vi "Employee_Lookup(py).vi"(0 "Badge Scan In(str)":string, 11 "error in (no error)":errorcluster, 12 "Enable(t)":bool) -> (2 "standard output":string, 3 "Success?(t)":bool, 15 "error out":errorcluster)   [LabVIEW 2018]
uses:
  <vilib>/Utility/error.llb/DialogType.ctl
  Initialize References/Sequence Globals.vi
panel:
  out "py path":path
  out "Badge Scan Out(str)":string
  in  "ByPass(t)":bool
  out "SwExists?(t)":bool
  out "NameMatch?(t)":bool
  out "BadgeName":string
  out "DbName":string
  out "EmpNumMatch?(t)":bool
  out "DataBaseError?(T)":bool
  out "standard error":string
  # "001, RICK QUINTAL, NBPT"
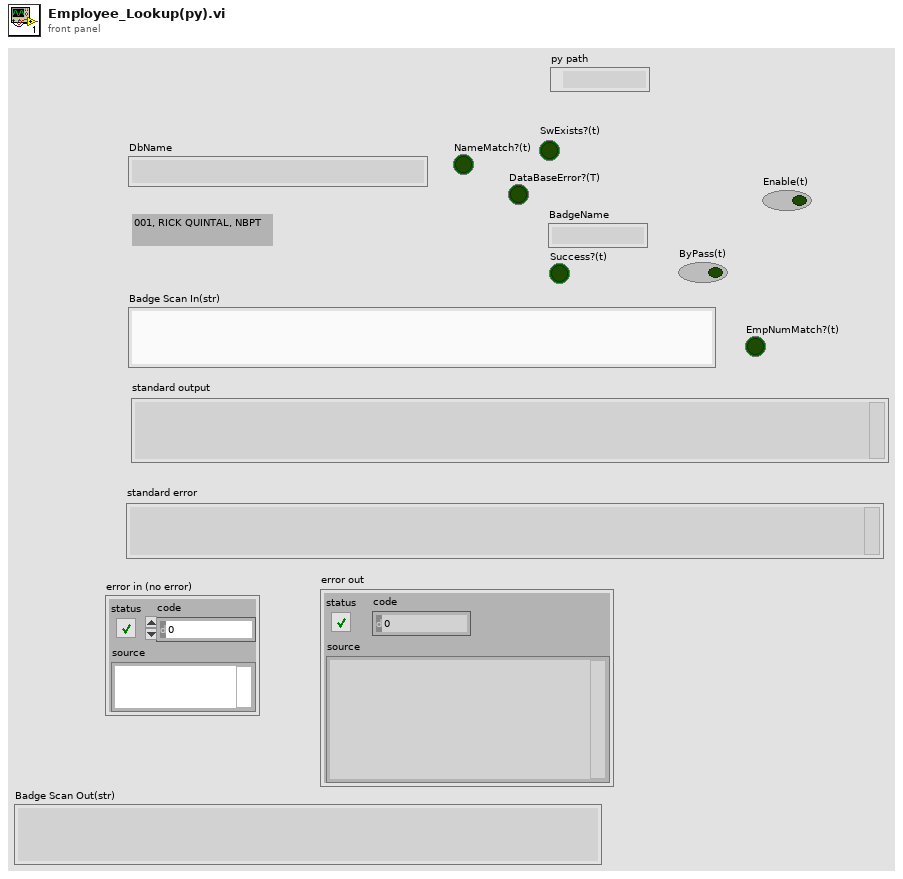
[diagram p1: front panel]
types:
  T1 = typedef "DialogType.ctl" = u16
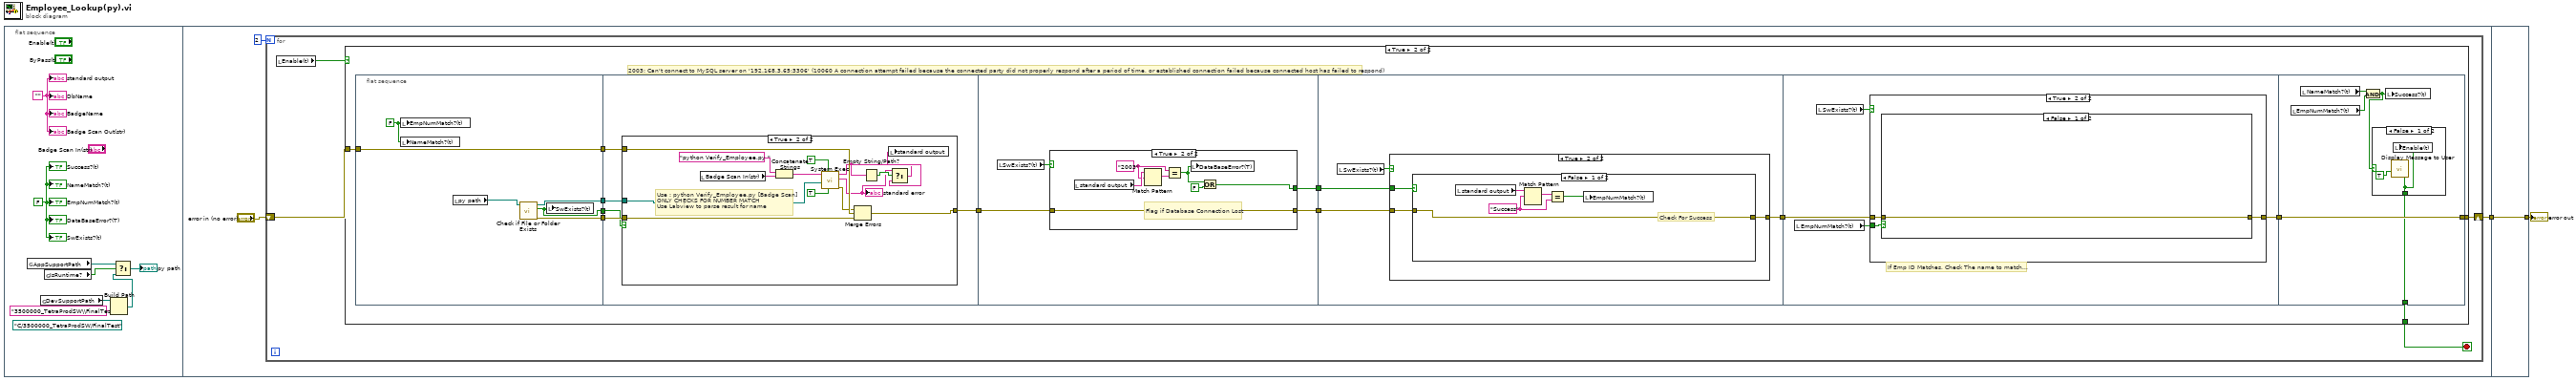
[diagram p0: block diagram]
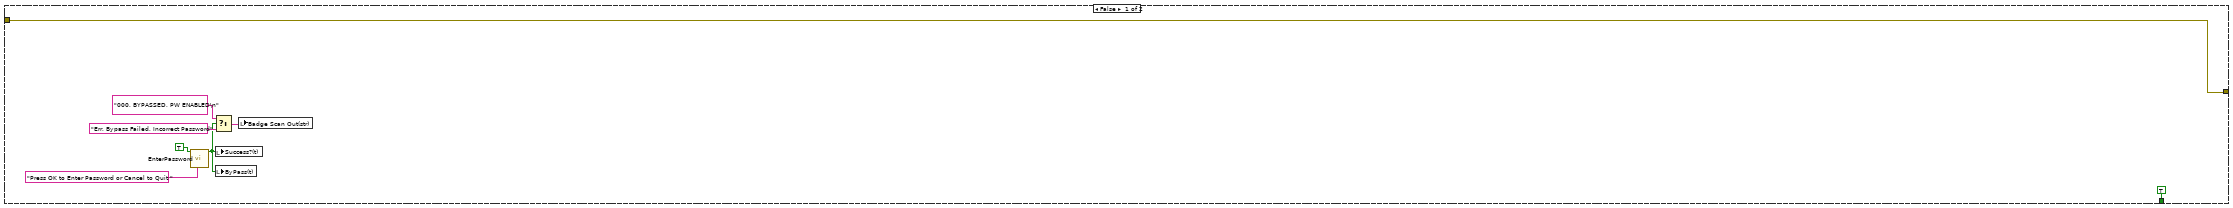
[diagram p2: hidden frame]
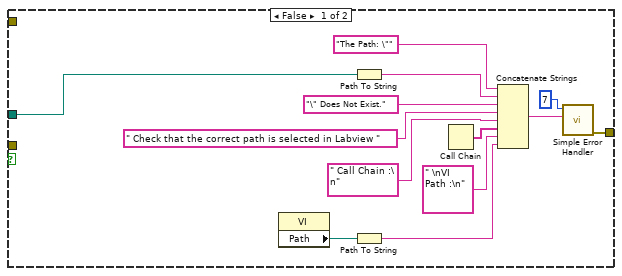
[diagram p3: hidden frame]
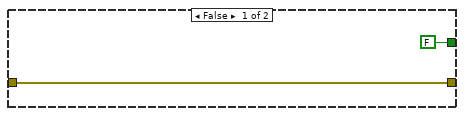
[diagram p4: hidden frame]
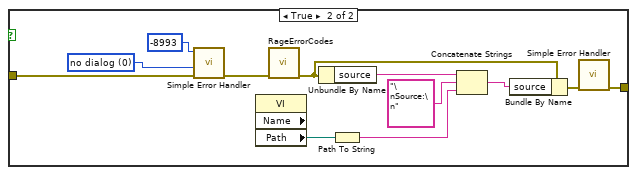
[diagram p6: hidden frame]
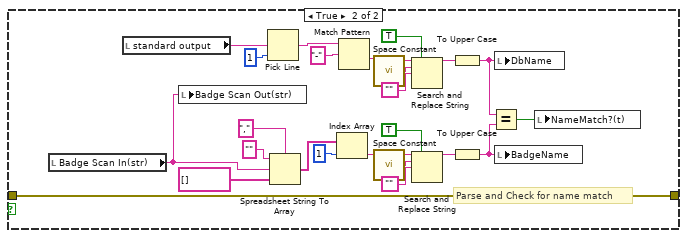
[diagram p8: hidden frame]
diagram:
  n1 = flat-sequence {
    tunnel: [w13] -> w1
    tunnel: [w155] -> w2
    tunnel: w1 -> [w155]
    frame #0 {
      (unwired) path "C:/3500000_TetraProdSW/FinalTest" ("working directory")
      w9 = ""
      w10 = FALSE ("Success?(t)")
      n2 = global read "Sequence Globals.vi" "AppSupportPath"() -> (w6:path)
      n3 = global read "Sequence Globals.vi" "DevSupportPath"() -> (w5:path)
      n4 = global read "Sequence Globals.vi" "IsRuntime?"() -> (w7:bool)
      n5 = Build Path(base path=w5, name or relative path="3500000_TetraProdSW\\FinalTest") -> (appended path=w3:path)
      n6 = Select(t=w6, s=w7, f=w3) -> (s? t:f=→"py path":path)
      "Success?(t)" <- w10
      "NameMatch?(t)" <- w10
      "EmpNumMatch?(t)" <- w10
      "DataBaseError?(T)" <- w10
      "SwExists?(t)" <- w10
      "standard output" <- w9
      "DbName" <- w9
      "BadgeName" <- w9
      "Badge Scan Out(str)" <- w9
    }
    frame #1 {
      n7 = for {
        N: 2 -> [_]
        shift-right: [w17] -> w13
        shift-left: "error in (no error)" -> [w16]
        stop <- w14 stop-if-true
        n8 = local read "Enable(t)"() -> (w15:bool)
        n9 = case shown="True" w15 {
          tunnel: [w25 w28] -> w17
          tunnel: w16 -> [w25 w27]
          tunnel: [TRUE ("OK") w26] -> w14
          frame False {
            n10 = call "EnterPassword.vi"("Message"="Press OK to Enter Password or Cancel to Quit ", "Enable(t)"=TRUE) -> ("success(t)"=w19:bool)  [unwired: 7 in, 2 out]
            n11 = Select(t="000, BYPASSED, PW ENABLED\n" ("Badge Scan(str)"), s=w19, f="Err, Bypass Failed, Incorrect Password") -> (s? t:f=w23:string)
            n12 = local write "Success?(t)"(w19) -> ()
            n13 = local write "ByPass(t)"(w19) -> ()
            n14 = local write "Badge Scan Out(str)"(w23) -> ()
          }
          frame True {
            # "2003: Can't connect to MySQL server on '192.168.3.65:3306' (10060 A connection attempt failed because the connected party did not properly respond after a period of time, or established connection failed because connected host has failed to respond)"
            n15 = flat-sequence {
              tunnel: [w40] -> w37
              tunnel: [w43] -> w36
              tunnel: [w42] -> w35
              tunnel: [w39] -> w34
              tunnel: w27 -> [w40]
              tunnel: [w47] -> w33
              tunnel: w37 -> [w48]
              tunnel: w36 -> [w46]
              tunnel: w35 -> [w45]
              tunnel: w34 -> [w44]
              tunnel: w33 -> [w76]
              tunnel: [w79] -> w32
              tunnel: [w77] -> w31
              tunnel: w32 -> [w90]
              tunnel: [w91] -> w30
              tunnel: w31 -> [w92]
              tunnel: w30 -> [w115]
              tunnel: [w116] -> w29
              tunnel: [w151] -> w28
              tunnel: w29 -> [w151]
              tunnel: [w147] -> w26
              frame #0 {
                w41 = FALSE ("NameMatch?(t)")
                n16 = local write "EmpNumMatch?(t)"(w41) -> ()
                n17 = local write "NameMatch?(t)"(w41) -> ()
                n18 = local read "py path"() -> (w38:path)
                n19 = call <vilib>:"Check if File or Folder Exists.vi"("path"=w38) -> ("error out"=w43:errorcluster, "file or folder exists?"=w39:bool, "dup path"=w42:path)  [unwired: 8 in]
                n20 = local write "SwExists?(t)"(w39) -> ()
              }
              frame #1 {
                n21 = case shown="True" w44 {
                  tunnel: w48 -> [_ w74]
                  tunnel: [w55 w75] -> w47
                  tunnel: w46 -> [_ w73]
                  tunnel: w45 -> [w61 w72]
                  frame False {
                    n22 = property class="VI"() -> ("Path"=w50:path)  [unwired: 2 in, 2 out]
                    n23 = Path To String(path=w61) -> (string=w60:string)
                    n24 = Path To String(path=w50) -> (string=w49:string)
                    n25 = Call Chain() -> (call chain=w53:string[])
                    n26 = Concatenate Strings("The Path: \"" ("string"), w60, "\" Does Not Exist." ("string"), " Check that the correct path is selected in Labview " ("string"), " Call Chain :\n" ("string"), w53, " \nVI Path :\n" ("string"), w49) -> (w54:string)
                    n27 = call <vilib>:"Simple Error Handler.vi"("error code (no error:0)"=7, "error source (\" \")"=w54) -> ("error out"=w55:errorcluster)  [unwired: 3 in, 4 out]
                  }
                  frame True {
                    # "Use : python Verify_Employee.py [Badge Scan]\nONLY CHECKS FOR NUMBER MATCH\nUse Labview to parse result for name"
                    n28 = local read "Badge Scan In(str)"() -> (w66:string)
                    n29 = Concatenate Strings("python Verify_Employee.py " ("command line"), w66) -> (w70:string)
                    n30 = call <vilib>:"System Exec.vi"("run minimized? (F)"=TRUE, "wait until completion? (T)"=TRUE, "working directory"=w72, "command line"=w70) -> ("error out"=w69:errorcluster, "standard error"=w64:string, "standard output"=w63:string)  [unwired: 4 in, 1 out]
                    "standard error" <- w64
                    n31 = Merge Errors(w69, w74, w73) -> (w75:errorcluster)
                    n32 = Empty String/Path?(string/path=w63) -> (empty?=w65:bool)
                    n33 = Select(t=w64, s=w65, f=w63) -> (s? t:f=w62:string)
                    n34 = local write "standard output"(w62) -> ()
                  }
                }
              }
              frame #2 {
                n35 = local read "SwExists?(t)"() -> (w78:bool)
                n36 = case shown="True" w78 {
                  tunnel: [FALSE w84] -> w79
                  tunnel: w76 -> [w80 w83]
                  tunnel: [w80 w83] -> w77
                  frame False {
                  }
                  frame True {
                    w85 = "2003" ("regular expression")
                    # "Flag if Database Connection Lost"
                    n37 = local read "standard output"() -> (w87:string)
                    n38 = Match Pattern(string=w87, regular expression=w85) -> (match substring=w88:string)  [unwired: 1 in, 3 out]
                    n39 = Equal?(x=w85, y=w88) -> (x = y?=w82:bool)
                    n40 = local write "DataBaseError?(T)"(w82) -> ()
                    n41 = Or(x=w82, y=FALSE) -> (x .or. y?=w84:bool)
                  }
                }
              }
              frame #3 {
                n42 = local read "SwExists?(t)"() -> (w89:bool)
                n43 = case shown="True" w89 {
                  tunnel: w92 -> [w93 w96]
                  tunnel: [w93 w95] -> w91
                  tunnel: w90 -> [_ w94]
                  frame False {
                  }
                  frame True {
                    n44 = case shown="False" w94 {
                      tunnel: w96 -> [w101 w112]
                      tunnel: [w101 w102] -> w95
                      frame False {
                        w98 = "Success" ("regular expression")
                        # "Check For Success"
                        n45 = local read "standard output"() -> (w100:string)
                        n46 = Match Pattern(string=w100, regular expression=w98) -> (match substring=w99:string)  [unwired: 1 in, 3 out]
                        n47 = Equal?(x=w99, y=w98) -> (x = y?=w97:bool)
                        n48 = local write "EmpNumMatch?(t)"(w97) -> ()
                      }
                      frame True {
                        w111 = T1 0 items=["no dialog", "OK message", "continue or stop message", "OK message + warnings", "continue/stop + warnings"] ("type of dialog (OK msg:1)")
                        n49 = call <vilib>:"Simple Error Handler.vi"("error code (no error:0)"=-8993, "type of dialog (OK msg:1)"=w111, "error in (no error)"=w112) -> ("error out"=w113:errorcluster)  [unwired: 2 in, 4 out]
                        n50 = property class="VI" props=["Name", "Path"]() -> ("Path"=w109:path)  [unwired: 2 in, 3 out]
                        n51 = call "RageErrorCodes.vi"("error in"=w113) -> ("error out"=w104:errorcluster)  [unwired: 8 in, 2 out]
                        n52 = Unbundle By Name(w104) -> ("source"=w108:string)
                        n53 = Path To String(path=w109) -> (string=w107:string)
                        n54 = Concatenate Strings(w108, "\nSource:\n" ("string"), w107) -> (w106:string)
                        n55 = Bundle By Name(cluster=w104, "source"=w106) -> (w103:errorcluster)
                        n56 = call <vilib>:"Simple Error Handler.vi"("error in (no error)"=w103) -> ("error out"=w102:errorcluster)  [unwired: 4 in, 4 out]
                      }
                    }
                  }
                }
              }
              frame #4 {
                # "If Emp ID Matches, Check The name to match..."
                n57 = local read "EmpNumMatch?(t)"() -> (w117:bool)
                n58 = local read "SwExists?(t)"() -> (w114:bool)
                n59 = case shown="True" w114 {
                  tunnel: w117 -> [_ w121]
                  tunnel: [w118 w120] -> w116
                  tunnel: w115 -> [w118 w119]
                  frame False {
                  }
                  frame True {
                    n60 = case shown="False" w121 {
                      tunnel: [w122 w127] -> w120
                      tunnel: w119 -> [w122 w127]
                      frame False {
                      }
                      frame True {
                        # "Parse and Check for name match"
                        n61 = local read "Badge Scan In(str)"() -> (w123:string)
                        n62 = local read "standard output"() -> (w146:string)
                        n63 = local write "Badge Scan Out(str)"(w123) -> ()
                        n64 = Pick Line(multi-line string=w146, line index=1) -> (output string=w144:string)  [unwired: 1 in]
                        n65 = Spreadsheet String To Array(delimiter (Tab)=",", format string="", spreadsheet string=w123, array type (2D Dbl)=string[] []) -> (array=w134:string[])
                        n66 = Index Array(array=w134, index=1) -> (element=w132:string)
                        n67 = Match Pattern(string=w144, regular expression="-") -> (after substring=w141:string)  [unwired: 1 in, 3 out]
                        n68 = call <vilib>:"Space Constant.vi"() -> ("String"=w140:string)
                        n69 = call <vilib>:"Space Constant.vi"() -> ("String"=w130:string)
                        n70 = Search and Replace String(replace all?=TRUE ("replace all? (F)"), input string=w141, search string=w140, replace string="") -> (result string=w138:string)  [unwired: 4 in, 3 out]
                        n71 = Search and Replace String(replace all?=TRUE ("replace all? (F)"), input string=w132, search string=w130, replace string="") -> (result string=w129:string)  [unwired: 4 in, 3 out]
                        n72 = To Upper Case(1:w138) -> (0:w125:string)
                        n73 = To Upper Case(1:w129) -> (0:w124:string)
                        n74 = Equal?(x=w125, y=w124) -> (x = y?=w126:bool)
                        n75 = local write "DbName"(w125) -> ()
                        n76 = local write "BadgeName"(w124) -> ()
                        n77 = local write "NameMatch?(t)"(w126) -> ()
                      }
                    }
                  }
                }
              }
              frame #5 {
                n78 = local read "EmpNumMatch?(t)"() -> (w149:bool)
                n79 = local read "NameMatch?(t)"() -> (w150:bool)
                n80 = And(x=w150, y=w149) -> (x .and. y?=w148:bool)
                n81 = case shown="False" w148 {
                  selector: w148 -> [_ w154]
                  tunnel: [w152 w154] -> w147
                  frame False {
                    n82 = call "Display Message to User"("Enable"=TRUE) -> ("OK"=w152:bool)  [unwired: 9 in, 1 out]
                    n83 = local write "Enable(t)"(w152) -> ()
                  }
                  frame True {
                  }
                }
                n84 = local write "Success?(t)"(w148) -> ()
              }
            }
          }
        }
      }
    }
    frame #2 {
    }
  }
  "error out" <- w2
